vi "Keep position above object.vi"(8 "bottom":dbl, 9 "right":dbl, 10 "top":dbl, 11 "left":dbl) -> (0 "Hover":bool, 1 "Roll":dbl, 2 "Pitch":dbl)   [LabVIEW 2014]
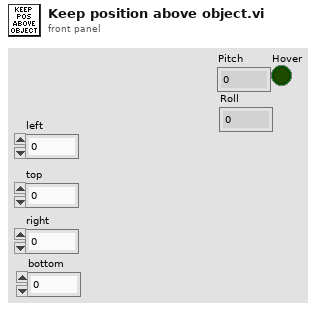
[diagram p1: front panel]
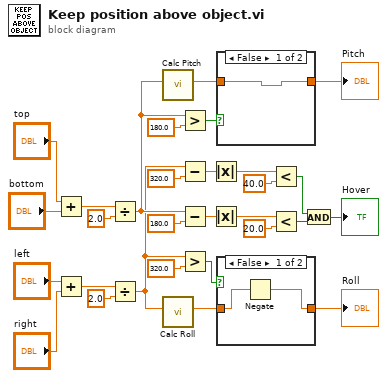
[diagram p0: block diagram]
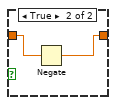
[diagram p3: hidden frame]
diagram:
  n1 = Add(x="top", y="bottom") -> (x+y=w23:dbl)
  n2 = Add(x="left", y="right") -> (x+y=w22:dbl)
  n3 = Divide(x=w23, y=2.0) -> (x/y=w12:dbl)
  n4 = Divide(x=w22, y=2.0) -> (x/y=w4:dbl)
  n5 = call "Calc Pitch.vi"("Position"=w12) -> ("Pitch"=w15:dbl)  [unwired: 10 in]
  n6 = call "Calc Roll.vi"("Position"=w4) -> ("Roll"=w14:dbl)  [unwired: 10 in]
  n7 = Greater?(x=w12, y=180.0) -> (0:w20:bool)
  n8 = Subtract(x=w4, y=320.0) -> (x-y=w8:dbl)
  n9 = Subtract(x=w12, y=180.0) -> (x-y=w13:dbl)
  n10 = Greater?(x=w4, y=320.0) -> (0:w18:bool)
  n11 = Absolute Value(x=w8) -> (abs(x)=w6:dbl)
  n12 = Absolute Value(x=w13) -> (abs(x)=w10:dbl)
  n13 = case shown="False" w20 {
    tunnel: w15 -> [w30 w32]
    tunnel: [w30 w31] -> w17
    frame False {
    }
    frame True {
      n14 = Negate(x=w32) -> (-x=w31:dbl)
    }
  }
  "Pitch" <- w17
  n15 = case shown="False" w18 {
    tunnel: w14 -> [w34 w35]
    tunnel: [w33 w35] -> w16
    frame False {
      n16 = Negate(x=w34) -> (-x=w33:dbl)
    }
    frame True {
    }
  }
  "Roll" <- w16
  n17 = Less?(x=w6, y=40.0) -> (x < y?=w3:bool)
  n18 = Less?(x=w10, y=20.0) -> (x < y?=w2:bool)
  n19 = And(x=w3, y=w2) -> (x .and. y?=→"Hover":bool)
